vi "GlobalVal.vi"() -> ()   [LabVIEW 2018]
panel:
  out "Battery":dbl(slide) scale=0.0..10.0
  in  "Photovoltaic":dbl(knob) scale=0.0..10.0
  out "GasLevel 2":dbl
  out "GasLevel 1":dbl
  out "Ki":dbl
  out "Kp":dbl
  out "tP":dbl
  out "kP":dbl
  out "tf":dbl
  out "kf":dbl
  out "OPC Server URL":string
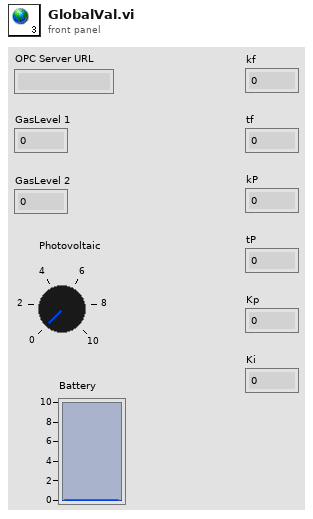
[diagram p1: front panel]
diagram:
